vi "task.vi"   [LabVIEW 2016, in "斯坦道多参数.lvlib"]
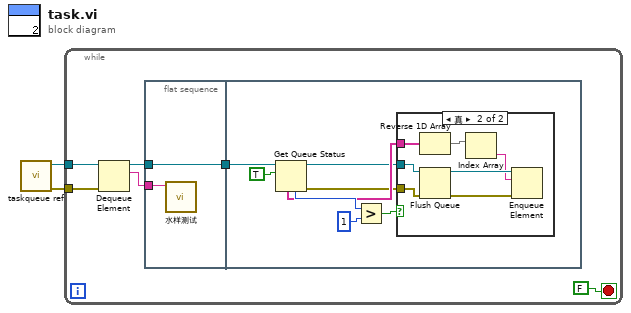
[diagram p0: block diagram]
diagram:
  n1 = call "taskqueue ref.vi"() -> ("错误输出"=w1:errorcluster, "队列输出"=w2:refnum<queue>)  [unwired: 10 in]
  n2 = while {
    tunnel: w2 -> [w8]
    tunnel: w1 -> [w7]
    stop <- FALSE stop-if-true
    n3 = Dequeue Element(queue=w8, error in (no error)=w7) -> (queue out=w3:refnum<queue>, element=w5:string)  [unwired: 1 in, 2 out]
    n4 = flat-sequence {
      tunnel: w5 -> [w10]
      tunnel: [w9] -> w4
      tunnel: w3 -> [w9]
      tunnel: w4 -> [w18]
      frame #0 {
        n5 = call "水样测试.vi"("数据标记表"=w10) -> ()  [unwired: 11 in]
      }
      frame #1 {
        n6 = Get Queue Status(queue=w18, return elements? (F)=TRUE ("返回元素？(F)")) -> (queue out=w12:refnum<queue>, error out=w11:errorcluster, # elements in queue=w16:i32, elements=w13:string[])  [unwired: 1 in, 4 out]
        n7 = Greater?(x=w16, y=1) -> (0:w14:bool)
        n8 = case shown="真" w14 {
          tunnel: w13 -> [_ w25]
          tunnel: w12 -> [_ w23]
          tunnel: w11 -> [_ w22]
          frame False {
          }
          frame True {
            n9 = Reverse 1D Array(array=w25) -> (reversed array=w24:string[])
            n10 = Flush Queue(queue=w23, error in (no error)=w22) -> (queue out=w21:refnum<queue>, error out=w19:errorcluster)  [unwired: 1 out]
            n11 = Index Array(array=w24) -> (element=w20:string)  [unwired: 1 in]
            n12 = Enqueue Element(queue=w21, element=w20, error in (no error)=w19) -> ()  [unwired: 1 in, 3 out]
          }
        }
      }
    }
  }
